vi "ELVIS III v1.0 Open Writing DMA.vi"(8 "error in (no error)":errorcluster) -> (0 "error out":errorcluster)   [LabVIEW 2021]
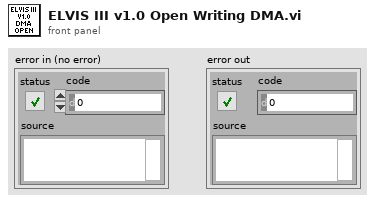
[diagram p1: front panel]
types:
  T1 = typedef "Block Write Resource.ctl" = refnum<vi>
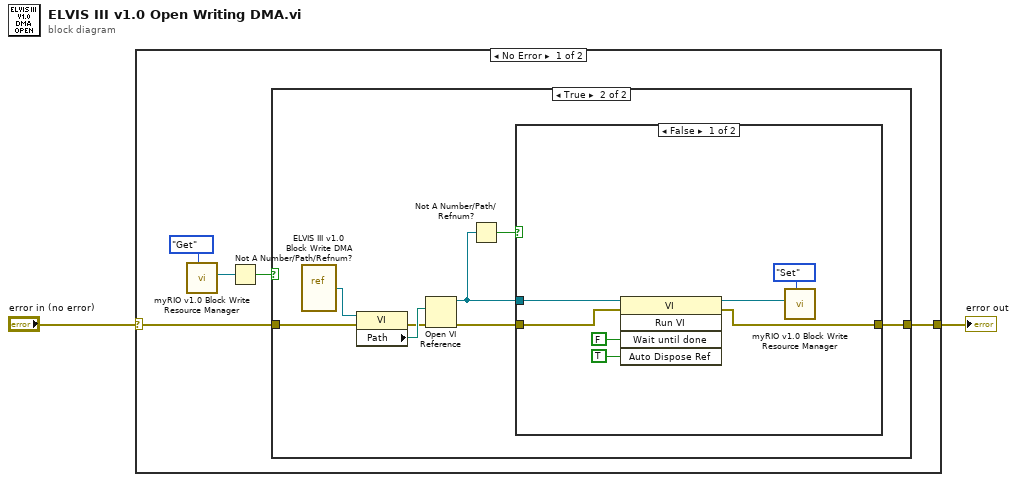
[diagram p0: block diagram]
diagram:
  n1 = case shown="No Error" "error in (no error)" {
    selector: "error in (no error)" -> [w4 w25]
    tunnel: [w7 w25] -> w2
    frame No Error {
      n2 = call <vilib>:"myRIO v1.0 Block Write Resource Manager.vi"("Action"=enum16{"Get", "Set", "Reset"}."Get" ("Enum")) -> ("Resource Data Out"=w3:T1)  [unwired: 10 in]
      n3 = Not A Number/Path/Refnum?(number/path/refnum=w3) -> (NaN/Path/Refnum?=w5:bool)
      n4 = case shown="True" w5 {
        tunnel: [w8 w9] -> w7
        tunnel: w4 -> [w8 w13]
        frame False {
        }
        frame True {
          n5 = vi-ref <vilib>:"ELVIS III v1.0 Block Write DMA.vi"() -> (w16:refnum<vi>)
          n6 = property class="VI"(reference=w16, error in=w13) -> (error out=w14:errorcluster, "Path"=w15:path)  [unwired: 1 out]
          n7 = Open VI Reference(vi path=w15, error in (no error)=w14) -> (vi reference=w11:refnum<vi>, error out=w10:errorcluster)  [unwired: 4 in]
          n8 = Not A Number/Path/Refnum?(number/path/refnum=w11) -> (NaN/Path/Refnum?=w12:bool)
          n9 = case shown="False" w12 {
            tunnel: w11 -> [w22 _]
            tunnel: w10 -> [w21 w24]
            tunnel: [w18 w24] -> w9
            frame False {
              n10 = invoke class="VI" method="Run VI"(reference=w22, error in=w21, "Wait until done"=FALSE ("Wait Until Done"), "Auto Dispose Ref"=TRUE ("Auto Dispose Reference")) -> (reference out=w17:refnum<vi>, error out=w18:errorcluster)  [unwired: 1 in, 3 out]
              n11 = call <vilib>:"myRIO v1.0 Block Write Resource Manager.vi"("Action"=enum16{"Get", "Set", "Reset"}."Set" ("Enum"), "Resource Data In"=w17) -> ()  [unwired: 9 in, 1 out]
            }
            frame True {
              # "No error is thrown since the error will be generated by the Open node."
            }
          }
        }
      }
    }
    frame Error {
    }
  }
  "error out" <- w2
